vi "Create.vi"(8 "error in (no error)":errorcluster, 10 "EnQr":refnum<class "Message Enqueuer.lvclass">) -> (0 "error out":errorcluster, 3 "ConfigAPI out":refnum<class "ConfigAPI.lvclass">)   [LabVIEW 2020, in "Volatus.lvlib" / "ConfigAPI.lvclass"]
uses:
  ConfigAPI.lvclass
  ConfigAPI.lvclass/ConfigAPI.ctl
  <vilib>/ActorFramework/Message Enqueuer/Message Enqueuer.lvclass
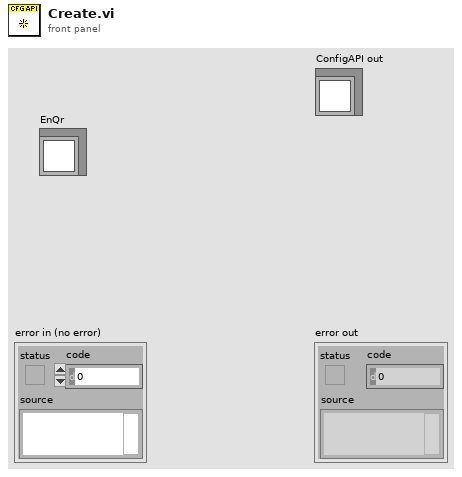
[diagram p1: front panel]
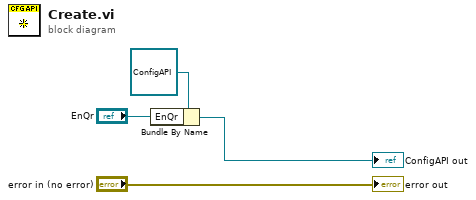
[diagram p0: block diagram]
diagram:
  n1 = Bundle By Name(cluster=refnum<class "ConfigAPI.lvclass"> refnum ("ConfigAPI in"), "EnQr"="EnQr") -> (→"ConfigAPI out":refnum<class "ConfigAPI.lvclass">)
  "error out" <- "error in (no error)"
